vi "HandleItemActivation.vi"(8 "error in (no error)":errorcluster, 11 "SystemExec in":refnum<class "SystemExec.lvclass">) -> (0 "error out":errorcluster, 3 "SystemExec out":refnum<class "SystemExec.lvclass">)   [LabVIEW 2009, in "NavScreen.lvlib" / "SystemExec.lvclass"]
uses:
  SystemExec.lvclass
  SystemExec.lvclass/SystemExec.ctl
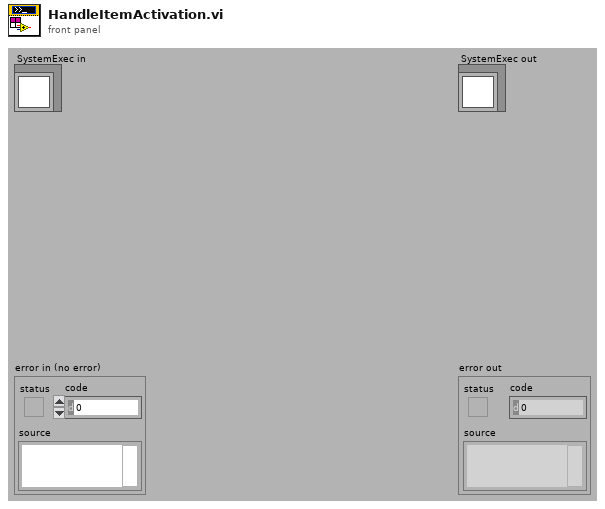
[diagram p1: front panel]
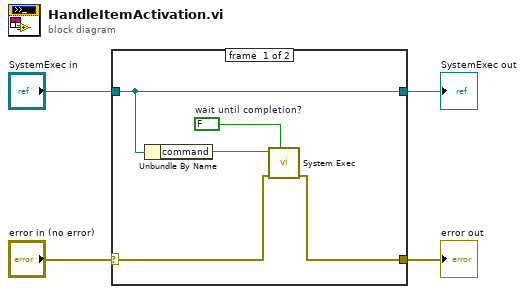
[diagram p0: block diagram]
diagram:
  n1 = case shown="No Error" "error in (no error)" {
    selector: "error in (no error)" -> [w8 w10]
    tunnel: "SystemExec in" -> [w5 w11]
    tunnel: [w7 w10] -> w2
    tunnel: [w5 w11] -> w1
    frame #0 {
      w6 = FALSE  # wait until completion?
      n2 = Unbundle By Name(w5) -> ("command"=w9:string)
      n3 = call <vilib>:"System Exec.vi"("wait until completion? (T)"=w6, "error in (no error)"=w8, "command line"=w9) -> ("error out"=w7:errorcluster)  [unwired: 5 in, 3 out]
    }
    frame #1 {
    }
  }
  "error out" <- w2
  "SystemExec out" <- w1
